vi "read.vi"() -> ()   [LabVIEW 2018]
panel:
  out "error out":T1
  in  "error in (no error)":T1
  out "connection reference 2":i16
  in  "connection reference":i16
  out "标准图像灰度阈值":T2={"10E-1Lux"=0.79900026, "10E-2Lux"=0.8030001, "10E-3Lux"=1.0, "10E-4Lux"=0.99999964} {"10E-4Lux" min=0 max=4 step=0.1 format="%.2f"; "10E-3Lux" min=0 max=4 step=0.01 format="%.2f"; "10E-1Lux" min=0 max=2 step=0.1 format="%.2f"; "10E-2Lux" min=0 max=2 step=0.1 format="%.2f"}
  out "faultthreshold":T3={"flickery_gray_thres"=8, "flash_gray_thres"=16, "light_gray_thres"=24, "black_gray_thres"=32, "flickery_size_thres"=33200, "flash_size_thres"=160, "light_size_thres"=16, "black_size_thres"=16}
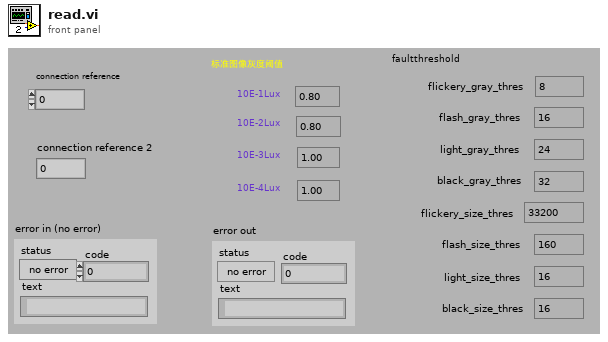
[diagram p1: front panel]
types:
  T1 = cluster{"status":bool, "code":i32, "text":string}
  T2 = cluster{"10E-1Lux":sgl, "10E-2Lux":sgl, "10E-3Lux":sgl, "10E-4Lux":sgl}
  T3 = cluster{"flickery_gray_thres":u8, "flash_gray_thres":u8, "light_gray_thres":u8, "black_gray_thres":u8, "flickery_size_thres":u32, "flash_size_thres":u32, "light_size_thres":u32, "black_size_thres":u32}
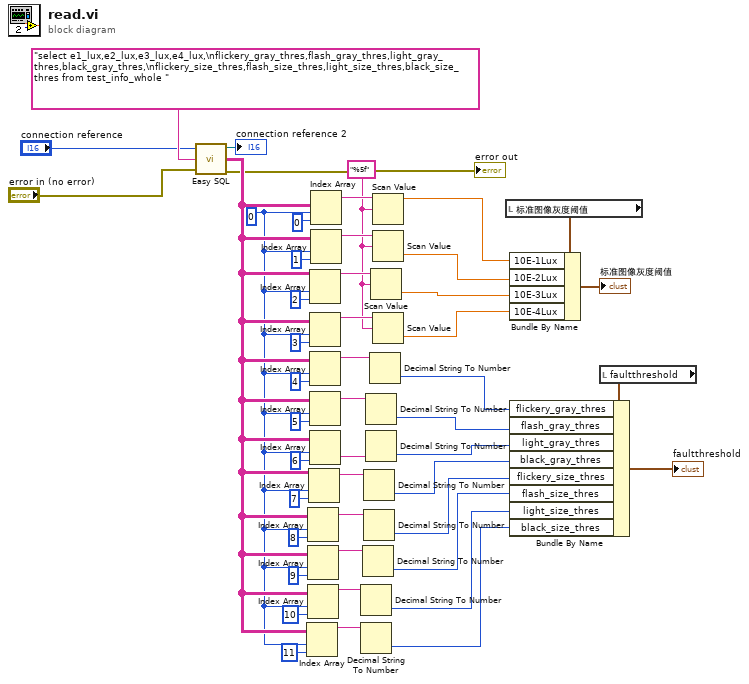
[diagram p0: block diagram]
diagram:
  w8 = "%5f"
  w45 = 0 ("Index")
  n1 = call <vilib>:"Easy SQL.vi"("connection"="connection reference", "SQL statement"="select e1_lux,e2_lux,e3_lux,e4_lux,\nflickery_gray_thres,flash_gray_thres,light_gray_thres,black_gray_thres,\nflickery_size_thres,flash_size_thres,light_size_thres,black_size_thres from test_info_whole ", "error in (no error)"="error in (no error)") -> ("connection"=→"connection reference 2":refnum<k7>, "error out"=→"error out":errorcluster, "query results"=w47:string[][])  [unwired: 2 out]
  n2 = Index Array(array=w47, index (row)=w45, index (col)=11 ("Index")) -> (element=w22:string)
  n3 = Index Array(array=w47, index (row)=w45, index (col)=8 ("Index")) -> (element=w25:string)
  n4 = Index Array(array=w47, index (row)=w45, index (col)=9 ("Index")) -> (element=w24:string)
  n5 = Index Array(array=w47, index (row)=w45, index (col)=10 ("Index")) -> (element=w23:string)
  n6 = Index Array(array=w47, index (row)=w45, index (col)=7 ("Index")) -> (element=w26:string)
  n7 = Index Array(array=w47, index (row)=w45, index (col)=2 ("Index")) -> (element=w31:string)
  n8 = Index Array(array=w47, index (row)=w45, index (col)=3 ("Index")) -> (element=w30:string)
  n9 = Index Array(array=w47, index (row)=w45, index (col)=4 ("Index")) -> (element=w29:string)
  n10 = Index Array(array=w47, index (row)=w45, index (col)=5 ("Index")) -> (element=w28:string)
  n11 = Index Array(array=w47, index (row)=w45, index (col)=6 ("Index")) -> (element=w27:string)
  n12 = Index Array(array=w47, index (row)=w45, index (col)=0) -> (element=w33:string)
  n13 = Index Array(array=w47, index (row)=w45, index (col)=1 ("Index")) -> (element=w32:string)
  n14 = Decimal String To Number(string=w23) -> (number=w18:i32)  [unwired: 2 in, 1 out]
  n15 = Decimal String To Number(string=w22) -> (number=w19:i32)  [unwired: 2 in, 1 out]
  n16 = Decimal String To Number(string=w24) -> (number=w17:i32)  [unwired: 2 in, 1 out]
  n17 = Decimal String To Number(string=w26) -> (number=w15:i32)  [unwired: 2 in, 1 out]
  n18 = Decimal String To Number(string=w25) -> (number=w16:i32)  [unwired: 2 in, 1 out]
  n19 = Decimal String To Number(string=w28) -> (number=w13:i32)  [unwired: 2 in, 1 out]
  n20 = Decimal String To Number(string=w27) -> (number=w14:i32)  [unwired: 2 in, 1 out]
  n21 = Decimal String To Number(string=w29) -> (number=w12:i32)  [unwired: 2 in, 1 out]
  n22 = Scan Value(string=w31, format string=w8) -> (value=w6:dbl)  [unwired: 1 in, 1 out]
  n23 = Scan Value(string=w33, format string=w8) -> (value=w9:dbl)  [unwired: 1 in, 1 out]
  n24 = Scan Value(string=w32, format string=w8) -> (value=w7:dbl)  [unwired: 1 in, 1 out]
  n25 = Scan Value(string=w30, format string=w8) -> (value=w5:dbl)  [unwired: 1 in, 1 out]
  n26 = local read "标准图像灰度阈值"() -> (w10:T2)
  n27 = Bundle By Name(cluster=w10, "10E-1Lux"=w9, "10E-2Lux"=w7, "10E-3Lux"=w6, "10E-4Lux"=w5) -> (→"标准图像灰度阈值":T2)
  n28 = local read "faultthreshold"() -> (w21:T3)
  n29 = Bundle By Name(cluster=w21, "flickery_gray_thres"=w12, "flash_gray_thres"=w13, "light_gray_thres"=w14, "black_gray_thres"=w15, "flickery_size_thres"=w16, "flash_size_thres"=w17, "light_size_thres"=w18, "black_size_thres"=w19) -> (→"faultthreshold":T3)
